vi "AMC Read Next Message.vi"(8 "error in (no error)":errorcluster, 9 "Termination List ([Exit])":string[](array[string])=["Exit"], 10 "timeout (1ms)":i32=1, 11 "Message Queue in":T3) -> (0 "error out":errorcluster, 1 "Message Value":string, 2 "Message Name":string, 3 "Message Queue out":T3, 4 "Message Attributes":T1, 5 "Exit Process":bool, 6 "Message":T2, 7 "Receiver Host":string)   [LabVIEW 2017]
doc: "This VI returns the next message from the message queue passed in. If the returned message matches any of the message names listed in the Termination List the Exit Process indicator will return True. If no message is available on the queue within the Timeout limit, the VI returns with the Timed Out indicator set True."
uses:
  subVIs/TypeDefs/amc_Message Queue.ctl
  subVIs/TypeDefs/amc_Message.ctl
  Tools/Keyed Array/Tools_KeyedArray KeyedArray.ctl
panel:
  out "Timed Out":bool
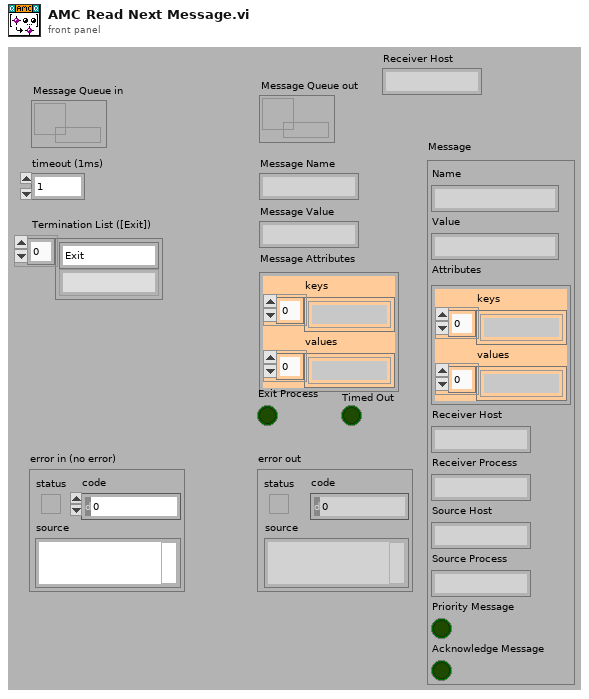
[diagram p1: front panel]
types:
  T1 = typedef "Tools_KeyedArray KeyedArray.ctl" = cluster{"keys":string[], "values":string[]}
  T2 = typedef "amc_Message.ctl" = cluster{"Name":string, "Value":string, "Attributes":T1, "Receiver Host":string, "Receiver Process":string, "Source Host":string, "Source Process":string, "Priority Message":bool, "Acknowledge Message":bool}
  T3 = typedef "amc_Message Queue.ctl" = refnum<queue>
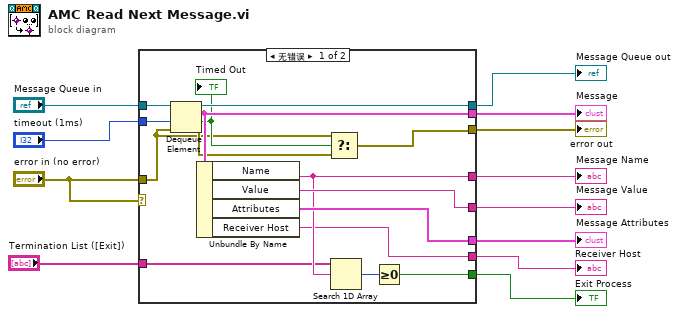
[diagram p0: block diagram]
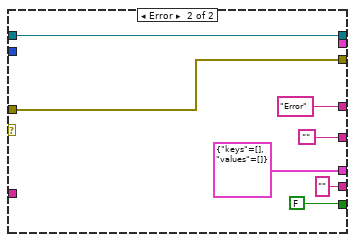
[diagram p2: hidden frame]
diagram:
  n1 = case shown="无错误" "error in (no error)" {
    tunnel: "Message Queue in" -> [w27 w34]
    tunnel: [w26 w34] -> w8
    tunnel: [w21 "Error"] -> w10
    tunnel: "error in (no error)" -> [w14 w32]
    tunnel: "timeout (1ms)" -> [w25 _]
    tunnel: [w15 w32] -> w9
    tunnel: [w23 ""] -> w7
    tunnel: [w24 _] -> w5
    tunnel: [w22 T1 {"keys"=[], "values"=[]} ("Attributes")] -> w4
    tunnel: "Termination List ([Exit])" -> [w20 _]
    tunnel: [w18 FALSE] -> w2
    tunnel: [w13 "" ("Receiver Host")] -> w1
    frame No Error {
      n2 = Dequeue Element(queue=w27, timeout in ms (-1)=w25, error in (no error)=w14) -> (queue out=w26:T3, element=w24:T2, timed out?=w17:bool, error out=w16:errorcluster)
      "Timed Out" <- w17
      n3 = Unbundle By Name(w24) -> ("Name"=w21:string, "Value"=w23:string, "Attributes"=w22:T1, "Receiver Host"=w13:string)
      n4 = Select(t=w14, s=w17, f=w16) -> (s? t:f=w15:errorcluster)
      n5 = Search 1D Array(1D array=w20, element=w21) -> (index of element=w19:i32)  [unwired: 1 out]
      n6 = Greater Or Equal To 0?(x=w19) -> (x >= 0?=w18:bool)
    }
    frame Error {
    }
  }
  "Message Queue out" <- w8
  "Message Name" <- w10
  "error out" <- w9
  "Message Value" <- w7
  "Message" <- w5
  "Message Attributes" <- w4
  "Exit Process" <- w2
  "Receiver Host" <- w1
